vi "Kaelus SWI Initialize.vi"(8 "error in (no error)":errorcluster, 11 "Configuration":T2={"BusType"=enum."USB", "Card"=0, "USB"="", "IP"=0, "COM"=1, "Baud Rate"=enum."9600"}) -> (0 "error out":errorcluster {"code" format="%.0x"}, 3 "DAQmx Dev Name (SWModule)":string, 5 "Kaelus SWI":T1)   [LabVIEW 2011]
uses:
  TypeDefs/Kaelus SWI Configuration.ctl
  TypeDefs/Kaelus SWI Instrument Info.ctl
  Summitek EXT/OpenG EXT/file/file.llb/File Exists - Scalar__ogtk.vi
  <vilib>/Utility/config.llb/Read Key (String).vi
  <vilib>/Utility/config.llb/NI_LVConfig.lvlib
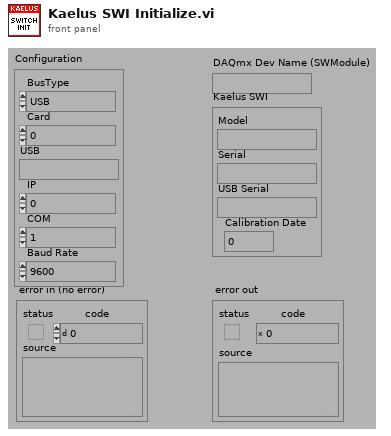
[diagram p1: front panel]
types:
  T1 = typedef "Kaelus SWI Instrument Info.ctl" = cluster{"Model":string, "Serial":string, "USB Serial":string, "Calibration Date":dbl}
  T2 = typedef "Kaelus SWI Configuration.ctl" = cluster{"BusType":enum32{"PCI/ISA/PCMCIA", "USB", "Ethernet", "Serial"}, "Card":i32, "USB":string, "IP":u32, "COM":i32, "Baud Rate":enum16{"300", "600", "1200", "2400", "4800", "9600"}}
  T3 = enum32{"invalid app kind", "Development System", "Run Time System", "Student Edition", "Embedded LabVIEW", "Evaluation", "Custom"}
  T4 = enum32{"PCI/ISA/PCMCIA", "USB", "Ethernet", "Serial"}
  T5 = enum16{"300", "600", "1200", "2400", "4800", "9600"}
  T6 = typedef "ModuleDef.ctl" = cluster{"DevName":string, "DevDetails":string, "DevID":u32, "HW Present":bool, "Module ID":u16, "ModuleCAL":path, "Module Type":T7, "Valid Cal?":bool, "UID":string}
  T7 = typedef "Module_Types.ctl" = enum16{"Unknown", "RF Module", "PA Module", "TR Module", "FE Module", "SW Module"}
  T8 = typedef "NI_LVConfig.lvlib/Config Data RefNum.ctl" = refnum<k1>
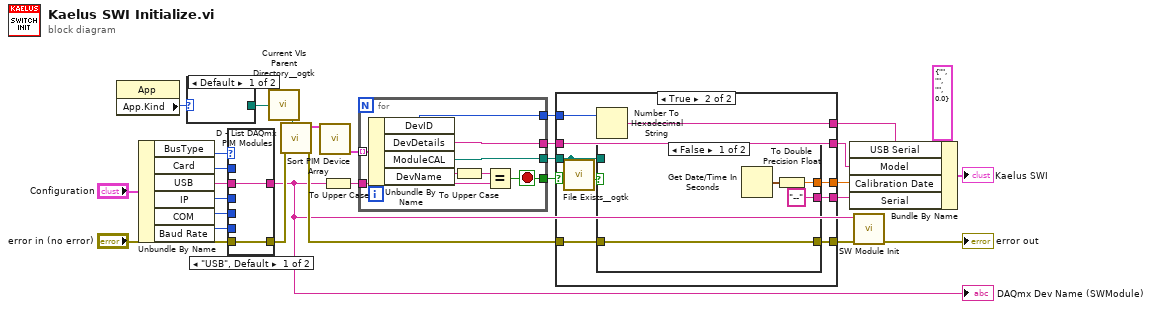
[diagram p0: block diagram]
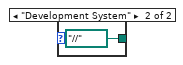
[diagram p2: hidden frame]
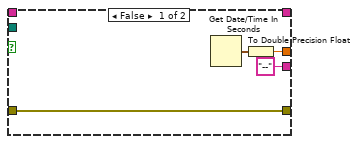
[diagram p3: hidden frame]
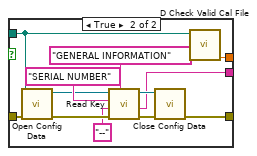
[diagram p4: hidden frame]
diagram:
  n1 = property class="App"() -> ("App.Kind"=w6:T3)  [unwired: 2 in, 2 out]
  n2 = Unbundle By Name("Configuration") -> ("BusType"=w28:T4, "Card"=w27:i32, "USB"=w26:string, "IP"=w25:u32, "COM"=w24:i32, "Baud Rate"=w22:T5)
  n3 = case shown="Default" w6 {
    tunnel: [_ path "../../.." ("Relative path (.)")] -> w5
    frame Default {
    }
    frame "Development System" {
    }
  }
  n4 = case shown="\"USB\", Default" w28 {
    tunnel: "error in (no error)" -> [w32 w33]
    tunnel: w27 -> [_ _]
    tunnel: w26 -> [w31 _]
    tunnel: w25 -> [_ _]
    tunnel: w24 -> [_ _]
    tunnel: [w32 w33] -> w17
    tunnel: [w31 _] -> w7
    tunnel: w22 -> [_ _]
    frame "USB", Default {
    }
    frame "PCI/ISA/PCMCIA", "Ethernet", "Serial" {
    }
  }
  "DAQmx Dev Name (SWModule)" <- w7
  n5 = call "Current VIs Parent Directory__ogtk.vi"("Relative path (.)"=w5) -> ("Parent Directory (+ Relative)"=w4:path)  [unwired: 4 in]
  n6 = call "D - List DAQmx PIM Modules.vi"("Cal Folder Path"=w4, "error in (no error)"=w17) -> ("error out"=w11:errorcluster, "PIM Modules"=w14:T6[])  [unwired: 8 in]
  n7 = call "Sort PIM Device Array.vi"("PIM Devices"=w14) -> ("SW Devices"=w13:T6[])  [unwired: 8 in, 6 out]
  n8 = To Upper Case(1:w7) -> (0:w12:string)
  n9 = for {
    tunnel: w13 -> [w41] mode=indexing
    tunnel: w12 -> [w39]
    tunnel: [w37] -> w10
    tunnel: [w36] -> w8
    tunnel: [w35] -> w9
    tunnel: [w34] -> w2
    stop <- w35 stop-if-true
    n10 = Unbundle By Name(w41) -> ("DevID"=w34:u32, "DevDetails"=w36:string, "ModuleCAL"=w37:path, "DevName"=w40:string)
    n11 = To Upper Case(1:w40) -> (0:w38:string)
    n12 = Equal?(x=w38, y=w39) -> (x = y?=w35:bool)
  }
  n13 = case shown="True" w9 {
    tunnel: w11 -> [w45 w54]
    tunnel: [w45 w53] -> w15
    tunnel: w10 -> [_ w52]
    tunnel: ["--" ("value") w50] -> w20
    tunnel: [w42 w49] -> w3
    tunnel: w8 -> [_ w48]
    tunnel: [_ w48] -> w19
    tunnel: w2 -> [_ w47]
    tunnel: [_ w46] -> w1
    frame False {
      n14 = Get Date/Time In Seconds() -> (seconds since 1Jan1904=w43:timestamp)
      n15 = To Double Precision Float(number=w43) -> (double precision float=w42:dbl)
    }
    frame True {
      n16 = call-poly "File Exists__ogtk.vi"("file path"=w52) -> ("exists"=w51:bool)  [unwired: 6 in, 1 out]
      n17 = Number To Hexadecimal String(2:w47) -> (0:w46:string)  [unwired: 1 in]
      n18 = case shown="False" w51 {
        tunnel: w54 -> [w58 w66]
        tunnel: [w58 w63] -> w53
        tunnel: w52 -> [_ w60]
        tunnel: ["--" ("value") w62] -> w50
        tunnel: [w55 w59] -> w49
        frame False {
          n19 = Get Date/Time In Seconds() -> (seconds since 1Jan1904=w56:timestamp)
          n20 = To Double Precision Float(number=w56) -> (double precision float=w55:dbl)
        }
        frame True {
          n21 = call <vilib>:"Open Config Data.vi"("error in (no error)"=w66, "configuration file path"=w60) -> ("error out"=w68:errorcluster, "refnum"=w64:T8)  [unwired: 7 in, 1 out]
          n22 = call-poly <vilib>:"Read Key.vi"("section"="GENERAL INFORMATION", "error in (no error)"=w68, "default value"="--", "key"="SERIAL NUMBER", "refnum"=w64) -> ("error out"=w67:errorcluster, "value"=w62:string, "refnum out"=w65:T8)  [unwired: 1 in, 3 out]
          n23 = call <vilib>:"Close Config Data.vi"("error in (no error)"=w67, "refnum"=w65) -> ("error out"=w63:errorcluster)  [unwired: 8 in, 1 out]
          n24 = call "D Check Valid Cal File.vi"("Device Cal File Path"=w60) -> ("Cal Date"=w59:dbl)  [unwired: 10 out]
        }
      }
    }
  }
  n25 = Bundle By Name(cluster=T1 {"Model"="", "Serial"="", "USB Serial"="", "Calibration Date"=0.0} ("Kaelus SWI"), "USB Serial"=w1, "Model"=w19, "Calibration Date"=w3, "Serial"=w20) -> (→"Kaelus SWI":T1)
  n26 = call "SW Module Init.vi"("error in (no error)"=w15, "DAQmx Dev Name (SWModule)"=w7) -> ("error out"=→"error out":errorcluster)  [unwired: 5 out]
